vi "Logs.vi"(7 "Action (GetList)":T1=enum."GetList", 8 "error in (no error)":errorcluster, 10 "Limit of logs":i32, 11 "Logs":T2) -> (0 "error out":errorcluster, 3 "List of logs":string)   [LabVIEW 2020]
uses:
  #typedef_Log.ctl
  #typedef_LogsAction.ctl
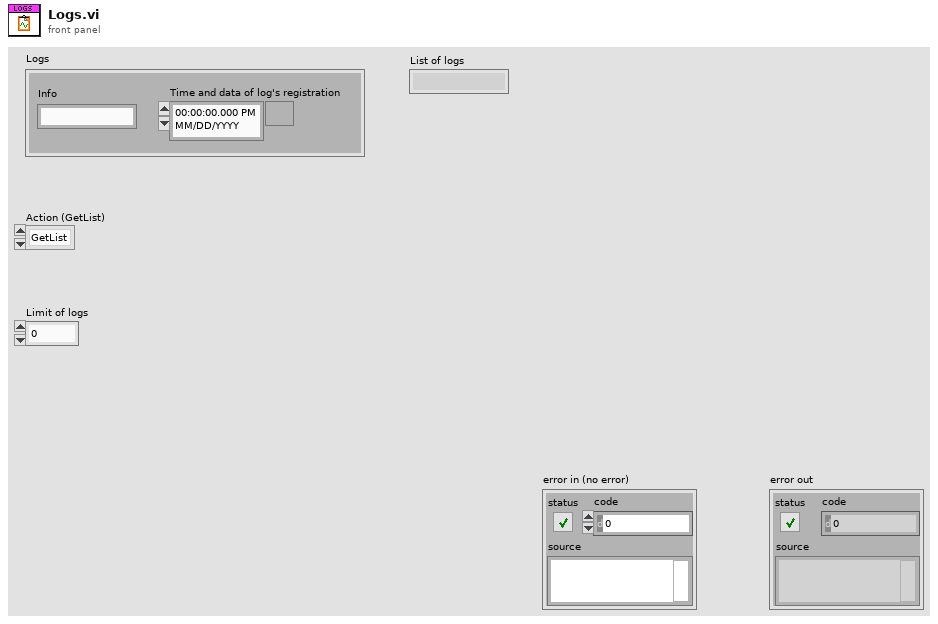
[diagram p1: front panel]
types:
  T1 = typedef "#typedef_LogsAction.ctl" = enum16{"ClearList", "AddRecord", "GetList"}
  T2 = typedef "#typedef_Log.ctl" = cluster{"Info":string, "Time and data of log's registration":timestamp}
  T3 = typedef "LVDateTimeRec.ctl" = cluster{"fractional second":dbl, "second":i32, "minute":i32, "hour":i32, "day of month":i32, "month":i32, "year":i32, "day of week":i32, "day of year":i32, "DST":i32}
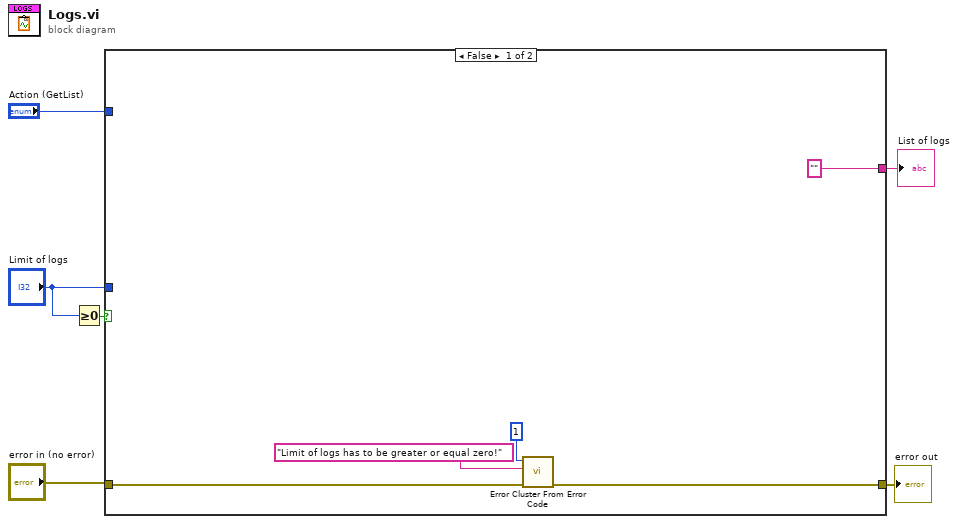
[diagram p0: block diagram]
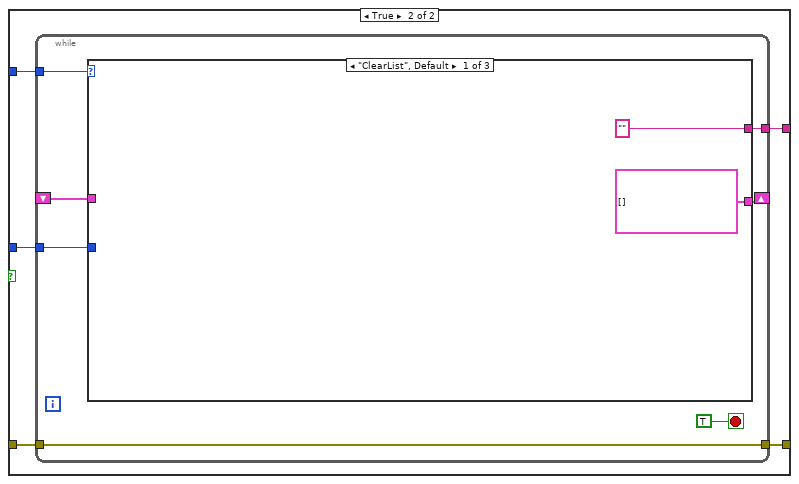
[diagram p2: hidden frame]
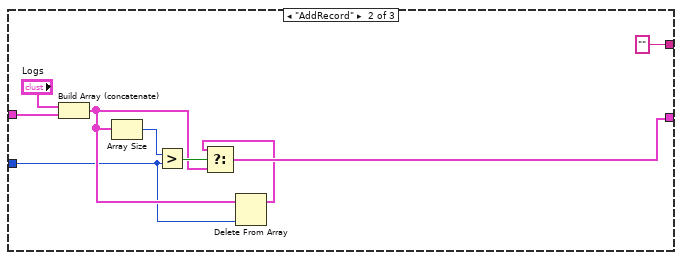
[diagram p3: hidden frame]
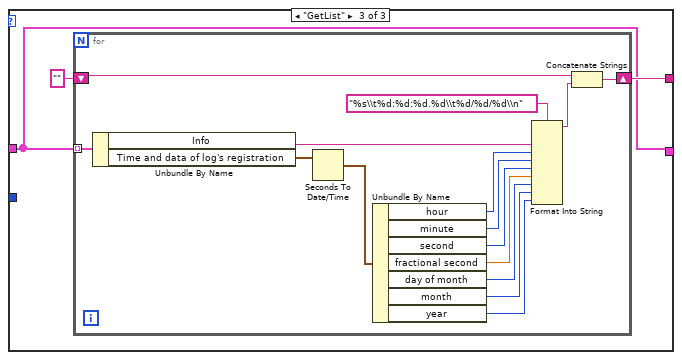
[diagram p4: hidden frame]
diagram:
  n1 = Greater Or Equal To 0?(x="Limit of logs") -> (x >= 0?=w3:bool)
  n2 = case shown="False" w3 {
    tunnel: ["" w16] -> w6
    tunnel: "Limit of logs" -> [_ w15]
    tunnel: "Action (GetList)" -> [_ w14]
    tunnel: "error in (no error)" -> [w9 w13]
    tunnel: [w8 w12] -> w1
    frame False {
      n3 = call <vilib>:"Error Cluster From Error Code.vi"("error in (no error)"=w9, "error message (\"\")"="Limit of logs has to be greater or equal zero!" ("error message (\"\")"), "error code (0)"=1) -> ("error out"=w8:errorcluster)  [unwired: 6 in]
    }
    frame True {
      n4 = while {
        tunnel: w14 -> [w22]
        shift-right: [w20] -> _
        shift-left: _ -> [w21]
        tunnel: w15 -> [w19]
        tunnel: [w18] -> w16
        tunnel: w13 -> [w17]
        tunnel: [w17] -> w12
        stop <- TRUE stop-if-true
        n5 = case shown="\"ClearList\", Default" w22 {
          tunnel: w21 -> [_ w33 w36]
          tunnel: [T2[] [] w31 w36] -> w20
          tunnel: w19 -> [_ w27 _]
          tunnel: ["" "" w37] -> w18
          frame "ClearList", Default {
          }
          frame "AddRecord" {
            n6 = Build Array (concatenate)("Logs", w33) -> (w30:T2[])
            n7 = Array Size(array=w30) -> (size(s)=w29:i32)
            n8 = Greater?(x=w29, y=w27) -> (0:w32:bool)
            n9 = Delete From Array(array=w30, index=w27) -> (array with subset deleted=w28:T2[])  [unwired: 1 in, 1 out]
            n10 = Select(t=w28, s=w32, f=w30) -> (s? t:f=w31:T2[])
          }
          frame "GetList" {
            n11 = for {
              tunnel: w36 -> [w52] mode=indexing
              shift-right: [w38] -> w37
              shift-left: "" -> [w40]
              n12 = Unbundle By Name(w52) -> ("Info"=w49:string, "Time and data of log's registration"=w51:timestamp)
              n13 = Seconds To Date/Time(time stamp (now)=w51) -> (date time rec=w50:T3)  [unwired: 1 in]
              n14 = Unbundle By Name(w50) -> ("hour"=w47:i32, "minute"=w46:i32, "second"=w45:i32, "fractional second"=w44:dbl, "day of month"=w43:i32, "month"=w42:i32, "year"=w41:i32)
              n15 = Format Into String(format string="%s\\t%d:%d:%d.%d\\t%d/%d/%d\\n", w49, w47, w46, w45, w44, w43, w42, w41) -> (resulting string=w39:string)  [unwired: 2 in, 1 out]
              n16 = Concatenate Strings(w40, w39) -> (w38:string)
            }
          }
        }
      }
    }
  }
  "List of logs" <- w6
  "error out" <- w1
